vi "CaseStructureExample.vi"() -> ()   [LabVIEW 2018]
panel:
  out "Number of Even Values in Array":dbl
  in  "Array":dbl[](array[numeric])=[1.0, 2.0, 3.0, 4.0, 5.0]
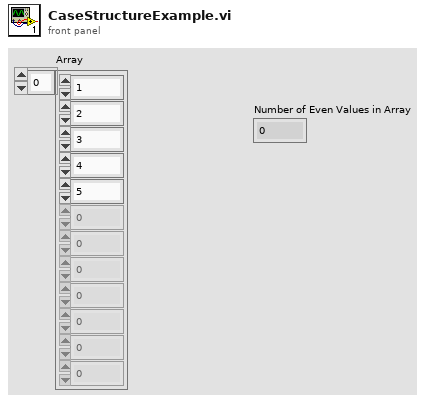
[diagram p1: front panel]
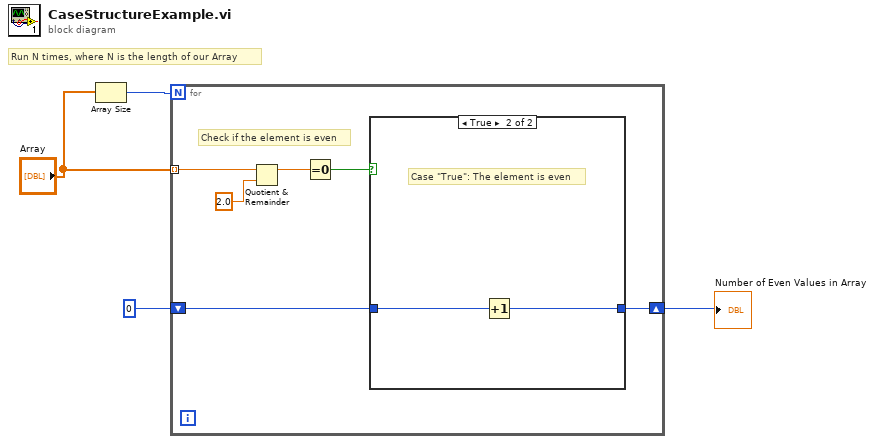
[diagram p0: block diagram]
diagram:
  # "Run N times, where N is the length of our Array"
  n1 = Array Size(array="Array") -> (size(s)=w4:i32)
  n2 = for {
    N: w4 -> [_]
    tunnel: "Array" -> [w9] mode=indexing
    shift-right: [w5] -> w1
    shift-left: 0 -> [w6]
    # "Check if the element is even"
    n3 = Quotient & Remainder(x=w9, y=2.0) -> (x-y*floor(x/y)=w8:dbl)  [unwired: 1 out]
    n4 = Equal To 0?(x=w8) -> (x = 0?=w10:bool)
    n5 = case shown="True" w10 {
      tunnel: w6 -> [w11 w13]
      tunnel: [w11 w12] -> w5
      frame False {
        # "Case \"False\": The element is odd"
      }
      frame True {
        # "Case \"True\": The element is even"
        n6 = Increment(x=w13) -> (x+1=w12:i32)
      }
    }
  }
  "Number of Even Values in Array" <- w1
